vi "datatest.vi"() -> ()   [LabVIEW 2012]
uses:
  <vilib>/Platform/TimedLoop/XDataNode/timing_clust.ctl
  <vilib>/Platform/TimedLoop/XDataNode/nitl_modes.ctl
  <vilib>/Platform/TimedLoop/XDataNode/wakeup.ctl
  <vilib>/Platform/TimedLoop/XDataNode/loadnilvce.vi
  <vilib>/Platform/TimedLoop/XDataNode/XDataNode.xnode
  <vilib>/Platform/TimedLoop/XDataNode/XDNodeRunTimeDep.lvlib
panel:
  in  "布尔":bool
  in  "停止":bool
  in  "status":u8
  in  "longitude":i32
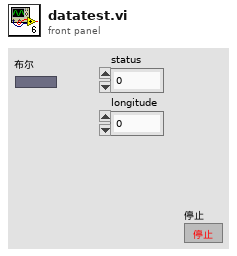
[diagram p1: front panel]
types:
  T1 = typedef "XDNodeRunTimeDep.lvlib/timing_clust.ctl" = cluster{"Expected End [f-1]":u64, "Actual End [f-1]":u64, "Finished Late? [f-1]":bool, "Expected End [i-1]":u64, "Actual End [i-1]":u64, "Finished Late? [i-1]":bool, "Expected Start [i]":u64, "Actual Start [i]":u64, "Expected Start [f]":u64, "Actual Start [f]":u64, "Source Name":string, "Structure Name":string, "Period":i64, "Deadline":i64, "Offset":i64, "Start":i64, "Priority":i32, "Timeout":i32, "Mode":T2, "Wakeup Reason":T3, "Error":errorcluster, "Source Type":string, "Secondary Source Type":string, "Global End Time":u64, "Global Start Time":u64, "Frame Duration":u64, "Iteration Duration":u64, "Assigned CPU":i32, "I/O Scan Engine Mode":u32}
  T2 = typedef "XDNodeRunTimeDep.lvlib/nitl_modes.ctl" = enum32{"No Change", "Process missed periods, maintain original phase", "Discard missed periods, maintain original phase", "Process missed periods, ignore original phase", "Discard missed periods, ignore original phase"}
  T3 = typedef "XDNodeRunTimeDep.lvlib/wakeup.ctl" = enum32{"Normal", "Aborted", "Asynchronous wakeup", "Timing source error", "Timed loop error", "Timeout"}
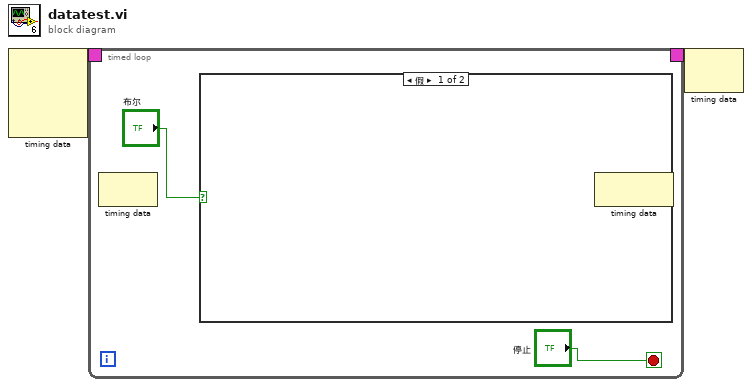
[diagram p0: block diagram]
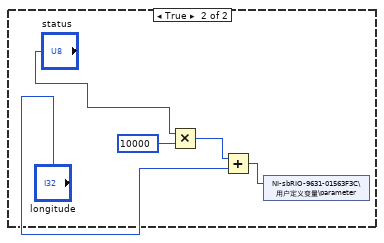
[diagram p2: hidden frame]
diagram:
  n1 = node-c288() -> (w2:T1)  [unwired: 4 in]
  n2 = timed-loop {
    timing: w2 -> [_]
    timing-out: [_] -> w1
    stop <- "停止" stop-if-true
    n3 = node-c288() -> ()  [unwired: 1 in, 1 out]
    n4 = case shown="假" "布尔" {
      frame False {
      }
      frame True {
        n5 = Multiply(x="status", y=10000) -> (x*y=w8:i32)
        n6 = Add(x=w8, y="longitude") -> (x+y=w7:i32)
        n7 = shared-variable "NI-sbRIO-9631-01563F3C\\用户定义变量\\parameter"(w7) -> ()  [unwired: 1 in, 1 out]
      }
    }
    n8 = node-c288() -> ()  [unwired: 1 in, 1 out]
  }
  n9 = node-c288(w1) -> ()  [unwired: 1 out]
